vi "SaveError txt file.vi"(1 "內容":string, 2 "異常碼":string) -> ()   [LabVIEW 2015]
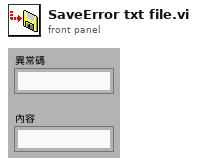
[diagram p1: front panel]
types:
  T1 = enum16{"open", "replace", "create", "open or create", "replace or create", "replace or create with confirmation"}
  T2 = typedef "LVDateTimeRec.ctl" = cluster{"fractional second":dbl, "second":i32, "minute":i32, "hour":i32, "day of month":i32, "month":i32, "year":i32, "day of week":i32, "day of year":i32, "DST":i32}
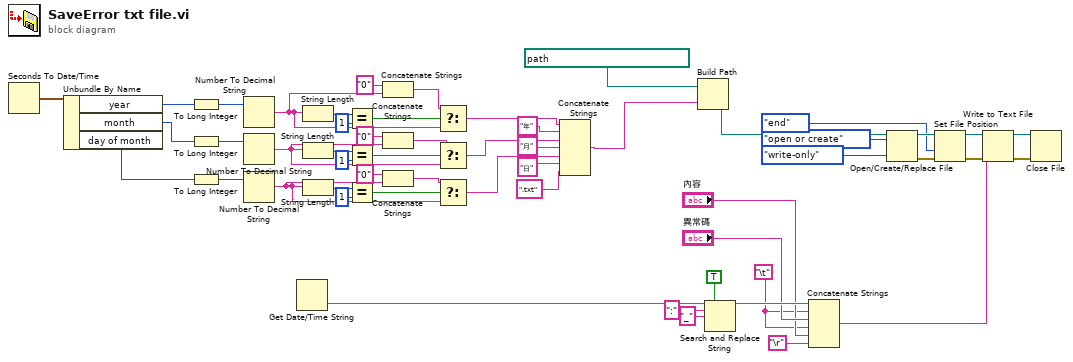
[diagram p0: block diagram]
diagram:
  w38 = "\t"
  n1 = Seconds To Date/Time() -> (date time rec=w33:T2)  [unwired: 2 in]
  n2 = Unbundle By Name(w33) -> ("year"=w32:i32, "month"=w28:i32, "day of month"=w9:i32)
  n3 = To Long Integer(number=w32) -> (32bit integer=w31:i32)
  n4 = To Long Integer(number=w28) -> (32bit integer=w30:i32)
  n5 = To Long Integer(number=w9) -> (32bit integer=w29:i32)
  n6 = Number To Decimal String(number=w31) -> (decimal integer string=w12:string)  [unwired: 1 in]
  n7 = Number To Decimal String(number=w30) -> (decimal integer string=w11:string)  [unwired: 1 in]
  n8 = Number To Decimal String(number=w29) -> (decimal integer string=w10:string)  [unwired: 1 in]
  n9 = Get Date/Time String() -> (time string=w43:string)  [unwired: 3 in, 1 out]
  n10 = String Length(string=w12) -> (length=w27:i32)
  n11 = String Length(string=w11) -> (length=w24:i32)
  n12 = String Length(string=w10) -> (length=w23:i32)
  n13 = Equal?(x=w27, y=1) -> (x = y?=w21:bool)
  n14 = Equal?(x=w24, y=1) -> (x = y?=w19:bool)
  n15 = Equal?(x=w23, y=1) -> (x = y?=w20:bool)
  n16 = Concatenate Strings("0" ("string"), w12) -> (w17:string)
  n17 = Concatenate Strings("0" ("string"), w11) -> (w15:string)
  n18 = Concatenate Strings("0" ("string"), w10) -> (w13:string)
  n19 = Select(t=w17, s=w21, f=w12) -> (s? t:f=w8:string)
  n20 = Select(t=w15, s=w19, f=w11) -> (s? t:f=w6:string)
  n21 = Select(t=w13, s=w20, f=w10) -> (s? t:f=w4:string)
  n22 = Concatenate Strings(w8, "年" ("replace string (\"\")"), w6, "月" ("replace string (\"\")"), w4, "日" ("string"), ".txt" ("string")) -> (w1:string)
  n23 = Build Path(base path=path "D:/半自動電檢機 Data/Error" ("appended path"), name or relative path=w1) -> (appended path=w35:path)
  n24 = Search and Replace String(replace all?=TRUE ("replace all? (F)"), input string=w43, search string=":", replace string="_" ("replace string (\"\")")) -> (result string=w45:string)  [unwired: 4 in, 3 out]
  n25 = Concatenate Strings(w45, w38, "異常碼", w38, "內容", "\r") -> (w37:string)
  n26 = Open/Create/Replace File(file path (use dialog)=w35, operation (0:open)=T1."open or create", access (0:read/write)=enum16{"read/write", "read-only", "write-only"}."write-only") -> (refnum out=w52:refnum<file>, error out=w50:errorcluster)  [unwired: 3 in, 1 out]
  n27 = Set File Position(refnum=w52, from (0:start)=enum16{"start", "end", "current"}."end", error in=w50) -> (refnum out=w48:refnum<file>, error out=w49:errorcluster)  [unwired: 1 in]
  n28 = Write to Text File(file (use dialog)=w48, text=w37, error in=w49) -> (refnum out=w46:refnum<file>, error out=w47:errorcluster)  [unwired: 1 in, 1 out]
  n29 = Close File(refnum=w46, error in=w47) -> ()  [unwired: 2 out]
